vi "Apply Effects.vi"(8 "error in (no error)":errorcluster, 10 "Instrument In":T2, 11 "MIDI Controls in":T1=variant(dbl 0.0)) -> (0 "error out":errorcluster, 2 "Instrument out":T2, 3 "MIDI Controls out":T1=variant(dbl 0.0))   [LabVIEW 2014, in "mySynthesizer.lvlib"]
uses:
  mySynthesizer.lvlib
  old/Instrument Level Processing/Instrument Level Processing.ctl
  old/MIDI Controls/MIDI Controls.ctl
  old/MIDI Controls/MIDI Controls.lvlib
  old/Instrument Level Processing/Instrument Level Processing.lvlib
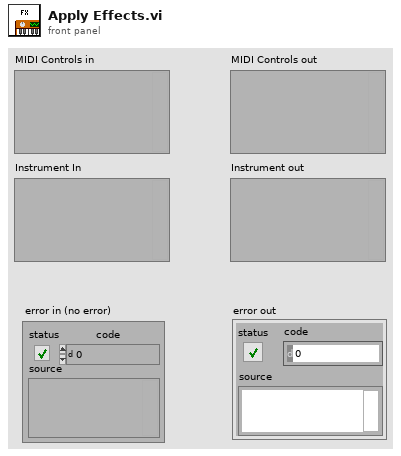
[diagram p1: front panel]
types:
  T1 = typedef "mySynthesizer.lvlib/MIDI Controls.lvlib/MIDI Controls.ctl" = variant
  T2 = typedef "mySynthesizer.lvlib/Instrument Level Processing.lvlib/Instrument Level Processing.ctl" = variant
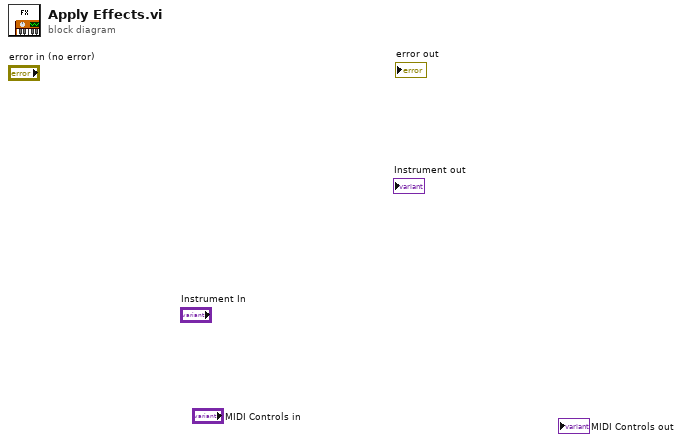
[diagram p0: block diagram]
diagram:
